vi "User_Database_Login_Confirm.vi"(8 "error in (no error)":errorcluster caption="Error In") -> (0 "error out":errorcluster caption="Error Out", 2 "User_Right":string, 3 "OK":bool)   [LabVIEW 2020]
uses:
  <vilib>/Utility/error.llb/whitespace.ctl
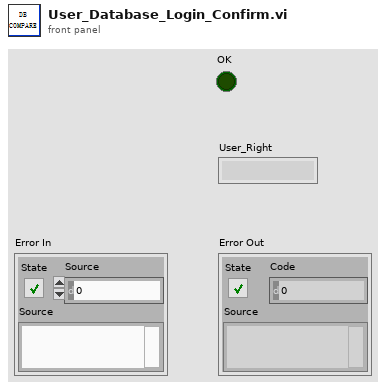
[diagram p1: front panel]
types:
  T1 = typedef "whitespace.ctl" = u16
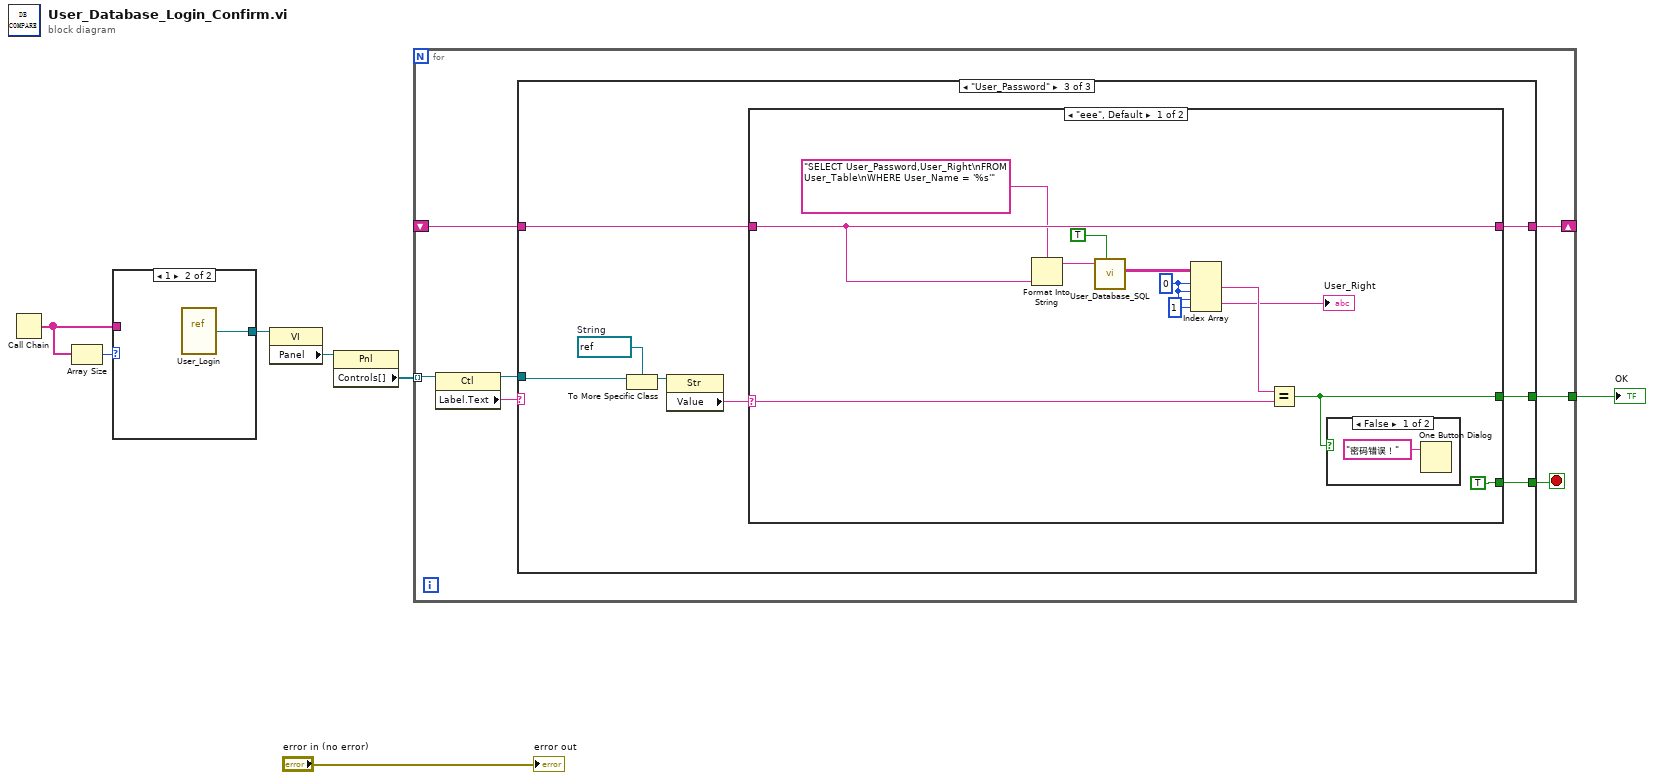
[diagram p0: block diagram]
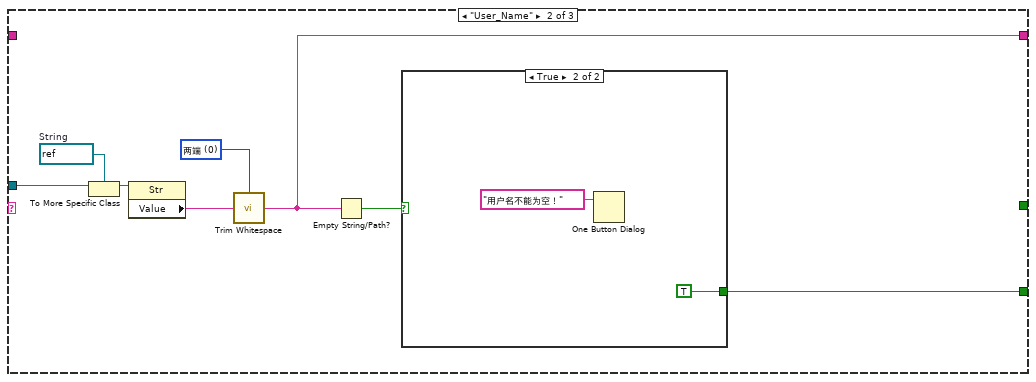
[diagram p3: hidden frame]
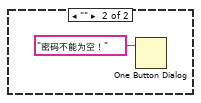
[diagram p6: hidden frame]
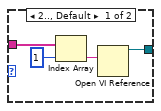
[diagram p7: hidden frame]
diagram:
  n1 = Call Chain() -> (call chain=w4:string[])
  n2 = Array Size(array=w4) -> (size(s)=w5:i32)
  n3 = case shown="1" w5 {
    tunnel: [w9 w12] -> w2
    tunnel: w4 -> [w8 _]
    frame 2.., Default {
      n4 = Index Array(array=w8, index=1 ("索引")) -> (element=w10:string)
      n5 = Open VI Reference(vi path=w10) -> (vi reference=w9:refnum<vi>)  [unwired: 5 in, 1 out]
    }
    frame 1 {
      n6 = vi-ref "User_Login.vi"() -> (w12:refnum<vi>)
    }
  }
  n7 = property class="VI"(reference=w2) -> ("Panel"=w3:refnum<vi>)  [unwired: 1 in, 2 out]
  n8 = property class="Pnl"(reference=w3) -> ("Controls[]"=w6:refnum<vi>[])  [unwired: 1 in, 2 out]
  n9 = for {
    tunnel: w6 -> [w19] mode=indexing
    shift-right: [w15] -> _
    shift-left: _ -> [w14]
    tunnel: [w13] -> w1
    stop <- w16 stop-if-true
    n10 = property class="Ctl"(reference=w19) -> (reference out=w17:refnum<vi>, "Label.Text"=w18:string)  [unwired: 1 in, 1 out]
    n11 = case shown="\"User_Password\"" w18 {
      tunnel: w17 -> [_ w28 w36]
      tunnel: [_ w23 w31] -> w16
      tunnel: [w20 w21 w32] -> w15
      tunnel: w14 -> [w20 _ w35]
      tunnel: [_ _ w33] -> w13
      frame "eee", Default {
      }
      frame "User_Name" {
        w25 = T1 0 items=["两端", "字符串首端", "字符串末端"] ("location (both)")
        w27 = refnum<vi> refnum  # String
        n12 = To More Specific Class(target class=w27, reference=w28) -> (specific class reference=w26:refnum<vi>)  [unwired: 1 in, 1 out]
        n13 = property class="Str"(reference=w26) -> ("Value"=w22:string)  [unwired: 1 in, 2 out]
        n14 = call <vilib>:"Trim Whitespace.vi"("string"=w22, "location (both)"=w25) -> ("trimmed string"=w21:string)
        n15 = Empty String/Path?(string/path=w21) -> (empty?=w24:bool)
        n16 = case shown="True" w24 {
          tunnel: [_ TRUE] -> w23
          frame False {
          }
          frame True {
            n17 = One Button Dialog(message="用户名不能为空！" ("消息")) -> ()  [unwired: 1 in, 1 out]
          }
        }
      }
      frame "User_Password" {
        w38 = refnum<vi> refnum  # String
        n18 = To More Specific Class(target class=w38, reference=w36) -> (specific class reference=w37:refnum<vi>)  [unwired: 1 in, 1 out]
        n19 = property class="Str"(reference=w37) -> ("Value"=w34:string)  [unwired: 1 in, 2 out]
        n20 = case shown="\"eee\", Default" w34 {
          selector: w34 -> [w50 _]
          tunnel: w35 -> [w49 _]
          tunnel: [w39 _] -> w33
          tunnel: [w49 _] -> w32
          tunnel: [TRUE _] -> w31
          frame "eee", Default {
            w42 = 0 ("索引 (行)")
            n21 = Format Into String(format string="SELECT User_Password,User_Right\nFROM User_Table\nWHERE User_Name = '%s'" ("SQL query"), w49) -> (resulting string=w46:string)  [unwired: 2 in, 1 out]
            n22 = call "User_Database_SQL.vi"("Get Record"=TRUE, "SQL query"=w46) -> ("Record"=w44:string[][])  [unwired: 7 in, 2 out]
            n23 = Index Array(array=w44, index (row) #1=w42, index (col) #1=w42, index (row) #2=w42, index (col) #2=1 ("禁用的索引 (列)")) -> (element #1=w43:string, element #2=→"User_Right":string)
            n24 = Equal?(x=w43, y=w50) -> (x = y?=w39:bool)
            n25 = case shown="False" w39 {
              frame False {
                n26 = One Button Dialog(message="密码错误！" ("消息")) -> ()  [unwired: 1 in, 1 out]
              }
              frame True {
              }
            }
          }
          frame "" {
            n27 = One Button Dialog(message="密码不能为空！" ("消息")) -> ()  [unwired: 1 in, 1 out]
          }
        }
      }
    }
  }
  "OK" <- w1
  "error out" <- "error in (no error)"
